vi "Main.vi"(8 "error in (no error)":errorcluster, 11 "Process in":refnum<class "Assembler.lvclass">) -> (0 "error out":errorcluster, 3 "Process out":refnum<class "Assembler.lvclass">)   [LabVIEW 2019, in "TimingDRV Engine.lvlib" / "Assembler.lvclass"]
uses:
  Assembler.lvclass
  C:/Users/XEnderMD/Desktop/CD Project Tools/Source/Engine/Windows/Parent Classes/Process/Process.lvclass
  Parent Classes/Process/Process.lvclass/Process.ctl
  Parent Classes/Process/Process.lvclass
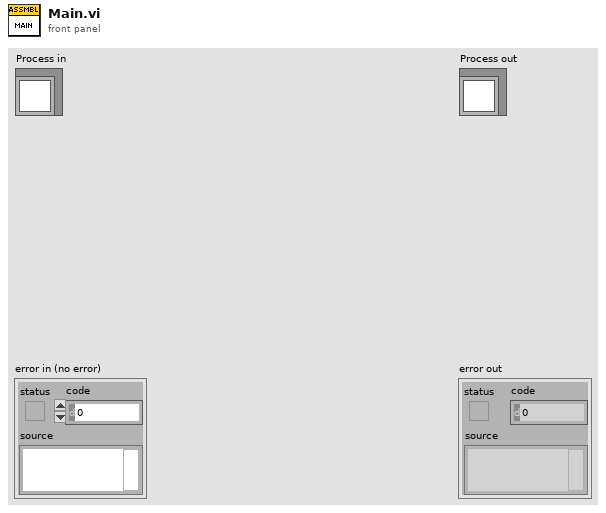
[diagram p1: front panel]
types:
  T1 = typedef "TimingDRV Engine.lvlib/Process.lvclass/Async Paramters.ctl" = cluster{"Device Reference":T2, "Device Clock":string, "Device Inputs FIFO":refnum<k33>, "Device Outputs FIFO":refnum<k33>, "CD Engine Event Ref":T3}
  T2 = typedef "Custom Device API.lvlib/Custom Device Item Ref.ctl" = u64
  T3 = typedef "Custom Device API.lvlib/Custom Device Engine Event Ref.ctl" = refnum<event-registration>
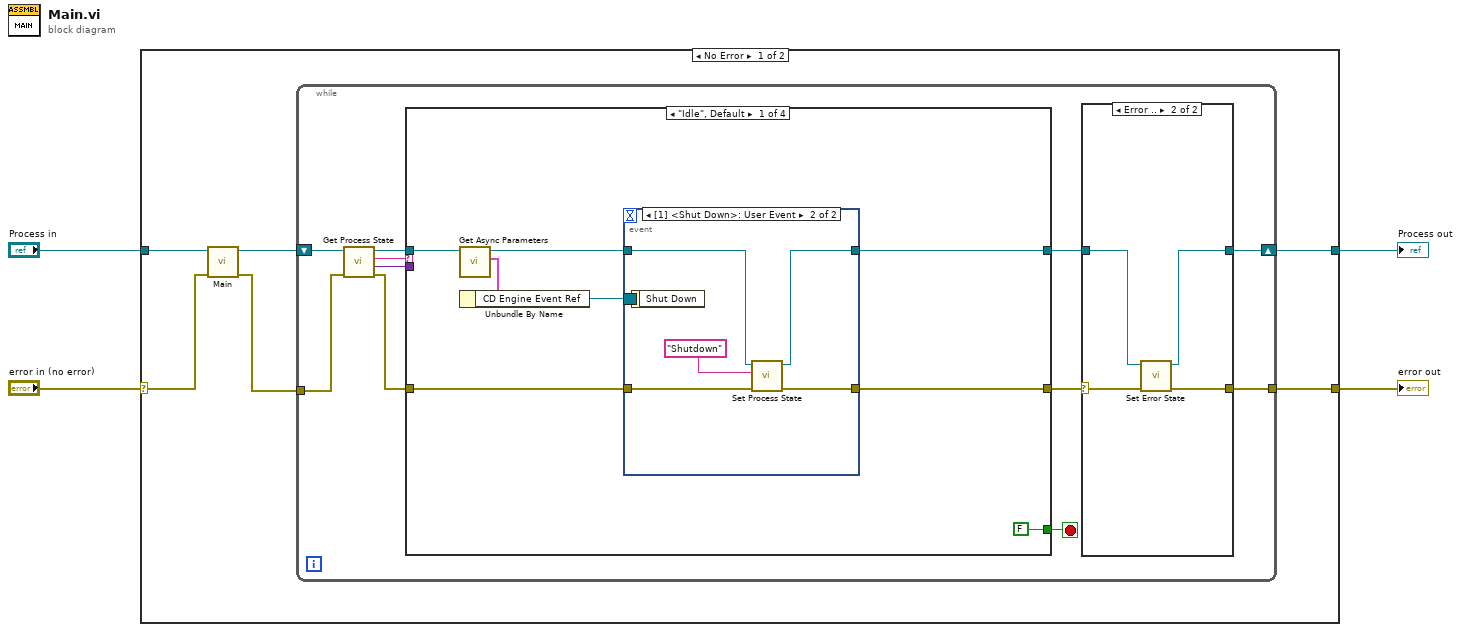
[diagram p0: block diagram]
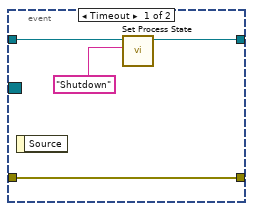
[diagram p3: hidden frame]
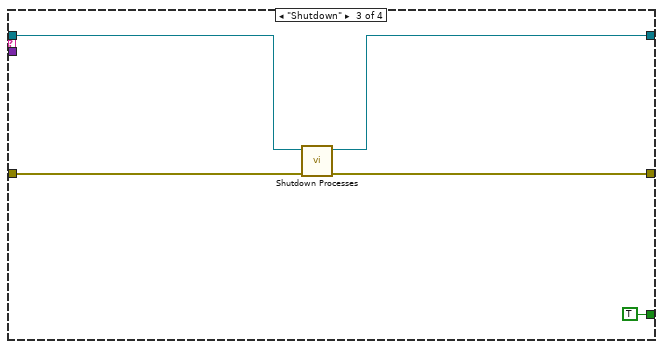
[diagram p5: hidden frame]
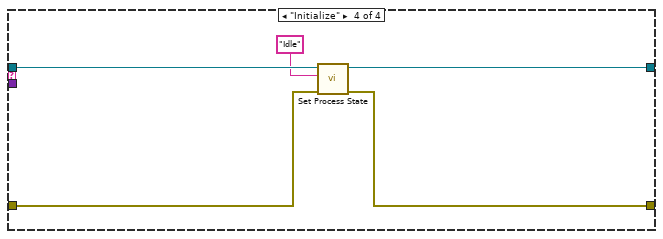
[diagram p6: hidden frame]
diagram:
  n1 = case shown="No Error" "error in (no error)" {
    selector: "error in (no error)" -> [w9 w58]
    tunnel: [w6 w58] -> w1
    tunnel: [w5 w57] -> w2
    tunnel: "Process in" -> [w10 w57]
    frame No Error {
      n2 = call-parent "Main.vi"("error in (no error)"=w9, "Process in"=w10) -> ("error out"=w7:errorcluster, "Process out"=w8:refnum<class "Assembler.lvclass">)  [unwired: 8 in]
      n3 = while {
        shift-right: [w13] -> w5
        shift-left: w8 -> [w20]
        tunnel: w7 -> [w21]
        tunnel: [w12] -> w6
        stop <- w11 stop-if-true
        n4 = call "Get Process State.vi"("error in (no error)"=w21, "Process in"=w20) -> ("error out"=w16:errorcluster, "Payload"=w17:variant, "Command"=w18:string, "Process out"=w19:refnum<class "Assembler.lvclass">)  [unwired: 6 in]
        n5 = case shown="\"Idle\", Default" w18 {
          tunnel: w19 -> [w31 w46 w49 w56]
          tunnel: w17 -> [_ _ _ _]
          tunnel: w16 -> [w33 w45 w50 w55]
          tunnel: [w34 w46 w48 w54] -> w15
          tunnel: [w32 w45 w47 w53] -> w14
          tunnel: [FALSE _ TRUE _] -> w11
          frame "Idle", Default {
            n6 = call "Get Async Parameters.vi"("Process in"=w31) -> ("Async Parameters"=w30:T1, "Process out"=w28:refnum<class "Assembler.lvclass">)  [unwired: 9 in]
            n7 = Unbundle By Name(w30) -> ("CD Engine Event Ref"=w29:T3)
            n8 = event shown="[1] <Shut Down>: User Event" {
              selector: w29 -> [_ _]
              dyn-events: _ -> [_ _]
              timeout: _ -> [_ _]
              tunnel: [w37 w42] -> w34
              tunnel: w33 -> [w39 w43]
              tunnel: [w39 w41] -> w32
              tunnel: w28 -> [w36 w40]
              event Timeout {
                n9 = event-data() -> ()  [unwired: 1 in, 1 out]
                n10 = call "Set Process State.vi"("Command"="Shutdown", "Process in"=w36) -> ("Process out"=w37:refnum<class "Assembler.lvclass">)  [unwired: 8 in, 1 out]
              }
              event User Event {
                n11 = event-data() -> ()  [unwired: 1 in, 1 out]
                n12 = call "Set Process State.vi"("error in (no error)"=w43, "Command"="Shutdown", "Process in"=w40) -> ("error out"=w41:errorcluster, "Process out"=w42:refnum<class "Assembler.lvclass">)  [unwired: 7 in]
              }
            }
          }
          frame "Error" {
          }
          frame "Shutdown" {
            n13 = call "Shutdown Processes.vi"("error in (no error)"=w50, "Assembler in"=w49) -> ("error out"=w47:errorcluster, "Assembler out"=w48:refnum<class "Assembler.lvclass">)  [unwired: 8 in]
          }
          frame "Initialize" {
            n14 = call "Set Process State.vi"("error in (no error)"=w55, "Command"="Idle", "Process in"=w56) -> ("error out"=w53:errorcluster, "Process out"=w54:refnum<class "Assembler.lvclass">)  [unwired: 7 in]
          }
        }
        n15 = case shown="Error .." w14 {
          selector: w14 -> [w22 w27]
          tunnel: w15 -> [w23 w26]
          tunnel: [w23 w25] -> w13
          tunnel: [w22 w24] -> w12
          frame No Error {
          }
          frame Error {
            n16 = call "Set Error State.vi"("error in (no error)"=w27, "Process in"=w26) -> ("error out"=w24:errorcluster, "Process out"=w25:refnum<class "Assembler.lvclass">)  [unwired: 8 in]
          }
        }
      }
    }
    frame Error {
    }
  }
  "error out" <- w1
  "Process out" <- w2
